vi "LaptopClient.vi"() -> ()   [LabVIEW 2018]
uses:
  Modes.ctl
  <vilib>/daq.io/MQTT LabVIEW Client/Controls/QoS.ctl
  <vilib>/daq.io/MQTT LabVIEW Client/Controls/DUP_Flag.ctl
  <vilib>/daq.io/MQTT LabVIEW Client/Controls/Retain_Flag.ctl
  <vilib>/daq.io/MQTT LabVIEW Client/Controls/Connect_Flags.ctl
  <vilib>/daq.io/MQTT LabVIEW Client/Controls/User_Info.ctl
  <vilib>/daq.io/MQTT LabVIEW Client/MQTT_Functions.lvlib
panel:
  out "Light":u16(ring)
  out "Fan":u16(ring)
  out "Reading Error":errorcluster
  out "Temperature":i32
  in  "Bulb":bool
  in  "Fan":bool
  in  "Mode Control":bool
  out "Mode":T1
  in  "stop":bool
  # "(auto)"
  # "(manual)"
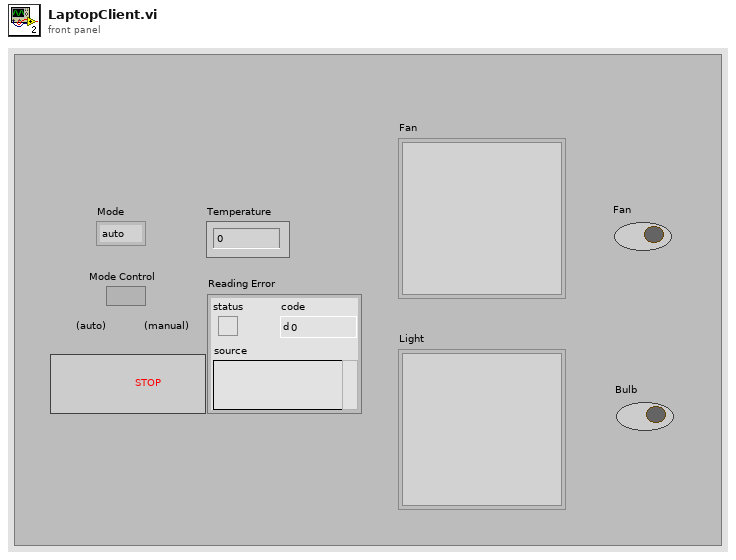
[diagram p1: front panel]
types:
  T1 = typedef "Modes.ctl" = enum16{"auto", "manual"}
  T2 = typedef "MQTT_Functions.lvlib/User_Info.ctl" = cluster{"User Name":string, "Password":string}
  T3 = typedef "MQTT_Functions.lvlib/QoS.ctl" = enum8{"At most once", "At least once", "Exactly once", "Reserved"}
  T4 = typedef "MQTT_Functions.lvlib/Connect_Flags.ctl" = cluster{"user name":bool, "password":bool, "will retain":bool, "will flag":bool, "clean session":bool, "reserved":bool, "will QoS":T3}
  T5 = typedef "MQTT_Functions.lvlib/DUP_Flag.ctl" = bool
  T6 = typedef "MQTT_Functions.lvlib/Retain_Flag.ctl" = bool
  T7 = cluster{"QoS":T3, "DUP":T5, "Retain":T6, "Keep Alive (sec)":u16}
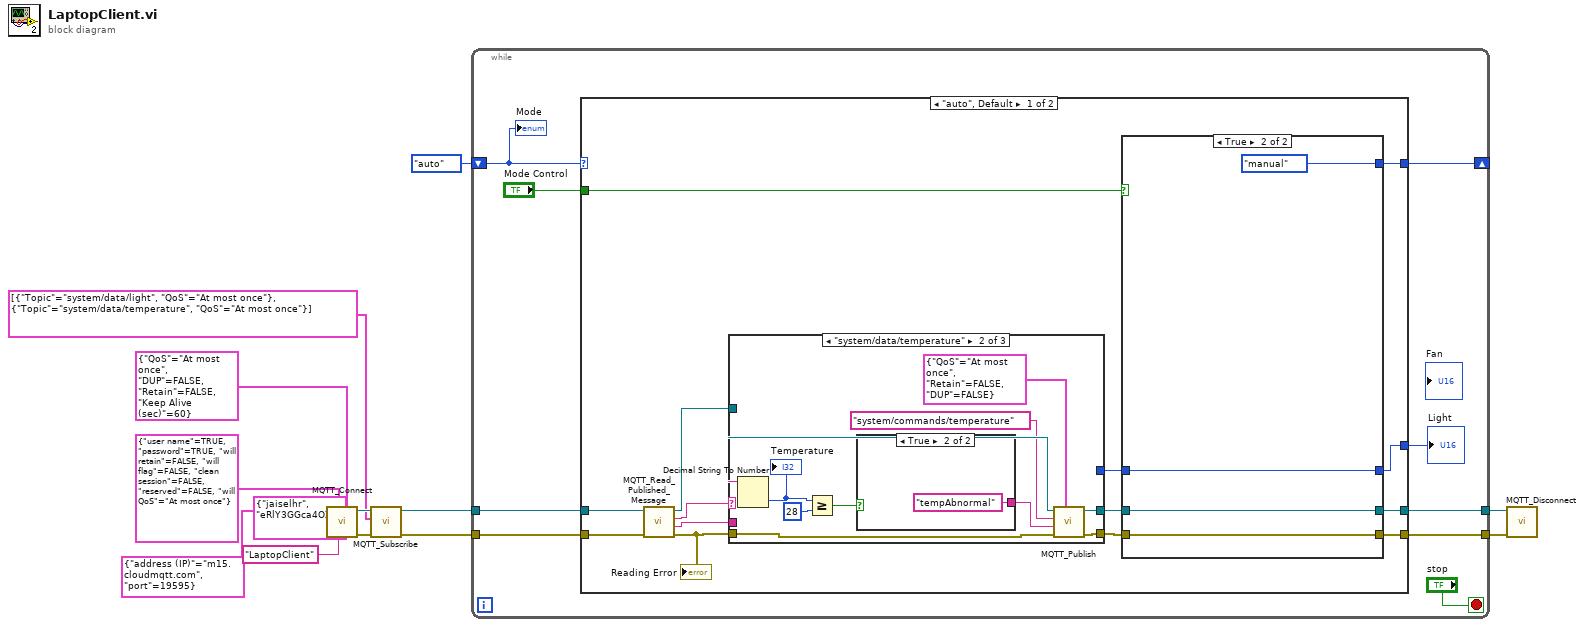
[diagram p0: block diagram]
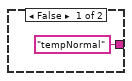
[diagram p3: hidden frame]
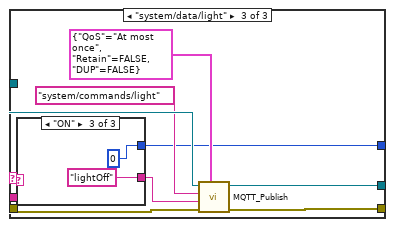
[diagram p4: hidden frame]
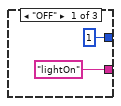
[diagram p5: hidden frame]
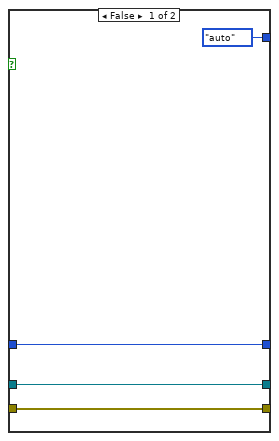
[diagram p7: hidden frame]
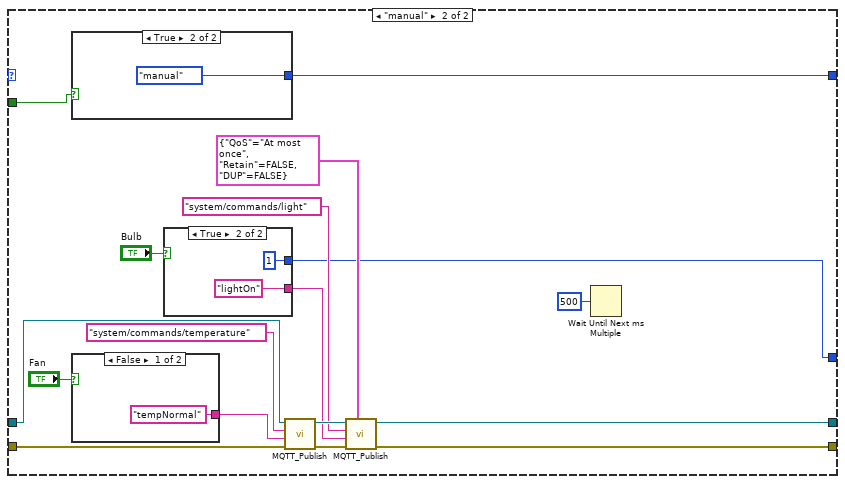
[diagram p8: hidden frame]
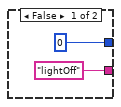
[diagram p9: hidden frame]
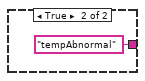
[diagram p10: hidden frame]
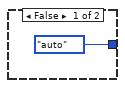
[diagram p11: hidden frame]
diagram:
  n1 = call <vilib>:"MQTT_Connect.vi"("Connect Meta"=T7 {"QoS"=enum."At most once", "DUP"=FALSE, "Retain"=FALSE, "Keep Alive (sec)"=60}, "Client ID"="LaptopClient", "Connect Flags"=T4 {"user name"=TRUE, "password"=TRUE, "will retain"=FALSE, "will flag"=FALSE, "clean session"=FALSE, "reserved"=FALSE, "will QoS"=enum."At most once"}, "User Info"=T2 {"User Name"="jaiselhr", "Password"="eRlY3GGca4OZ"}, "MQTT Broker"=cluster{"address (IP)":string, "port":u16} {"address (IP)"="m15.cloudmqtt.com", "port"=19595}) -> ("error out"=w7:errorcluster, "connection ID out"=w8:refnum<k5>)  [unwired: 4 in, 1 out]
  n2 = call <vilib>:"MQTT_Subscribe.vi"("error in (no error)"=w7, "Subscription Info Array"=cluster{"Topic":string, "QoS":T3}[] [{"Topic"="system/data/light", "QoS"=enum."At most once"}, {"Topic"="system/data/temperature", "QoS"=enum."At most once"}], "connection ID"=w8) -> ("error out"=w5:errorcluster, "connection ID out"=w4:refnum<k5>)  [unwired: 7 in]
  n3 = while {
    shift-right: [w21] -> _
    shift-left: Modes."auto" -> [w15]
    tunnel: w5 -> [w19]
    tunnel: w4 -> [w18]
    tunnel: [w17] -> w2
    tunnel: [w16] -> w3
    stop <- "stop" stop-if-true
    n4 = case shown="\"auto\", Default" w15 {
      tunnel: [w36 w88] -> w21
      tunnel: "Mode Control" -> [w35 w89]
      tunnel: w19 -> [w34 w84]
      tunnel: w18 -> [w33 w85]
      tunnel: [w26 w76] -> w17
      tunnel: [w25 w75] -> w16
      tunnel: [w23 w73] -> w14
      frame "auto", Default {
        n5 = call <vilib>:"MQTT_Read_Published_Message.vi"("error in (no error)"=w34, "connection ID"=w33) -> ("error out"=w30:errorcluster, "Message"=w31:string, "Topic Name"=w32:string, "connection ID out"=w28:refnum<k5>)  [unwired: 4 in, 2 out]
        "Reading Error" <- w30
        n6 = case shown="\"system/data/temperature\"" w32 {
          tunnel: w31 -> [_ w49 w60]
          tunnel: w30 -> [w38 w45 w59]
          tunnel: [w38 w44 w53] -> w29
          tunnel: w28 -> [w37 w41 w57]
          tunnel: [w37 w42 w56] -> w27
          tunnel: [_ _ w52] -> w24
          frame "False", Default {
          }
          frame "system/data/temperature" {
            n7 = Decimal String To Number(string=w49) -> (number=w48:i32)  [unwired: 2 in, 1 out]
            "Temperature" <- w48
            n8 = Greater Or Equal?(x=w48, y=28) -> (x >= y?=w46:bool)
            n9 = case shown="True" w46 {
              tunnel: ["tempNormal" ("Message to be published") "tempAbnormal" ("Message to be published")] -> w43
              frame False {
              }
              frame True {
              }
            }
            n10 = call <vilib>:"MQTT_Publish.vi"("Publish Meta"=cluster{"QoS":T3, "Retain":T6, "DUP":T5} {"QoS"=enum."At most once", "Retain"=FALSE, "DUP"=FALSE}, "error in (no error)"=w45, "Message to be published"=w43, "Topic"="system/commands/temperature", "connection ID"=w41) -> ("error out"=w44:errorcluster, "connection ID out"=w42:refnum<k5>)  [unwired: 5 in]
          }
          frame "system/data/light" {
            n11 = case shown="\"ON\"" w60 {
              tunnel: ["lightOn" ("Message to be published") _ "lightOff" ("Message to be published")] -> w58
              tunnel: [u16 1 ("Light") _ u16 0 ("Light")] -> w52
              frame "OFF" {
              }
              frame "", Default {
              }
              frame "ON" {
              }
            }
            n12 = call <vilib>:"MQTT_Publish.vi"("Publish Meta"=cluster{"QoS":T3, "Retain":T6, "DUP":T5} {"QoS"=enum."At most once", "Retain"=FALSE, "DUP"=FALSE}, "error in (no error)"=w59, "Message to be published"=w58, "Topic"="system/commands/light", "connection ID"=w57) -> ("error out"=w53:errorcluster, "connection ID out"=w56:refnum<k5>)  [unwired: 5 in]
          }
        }
        n13 = case shown="True" w35 {
          tunnel: [Modes."auto" ("Enum") Modes."manual" ("Enum")] -> w36
          tunnel: w29 -> [w66 w70]
          tunnel: w27 -> [w67 w71]
          tunnel: [w67 w71] -> w26
          tunnel: [w66 w70] -> w25
          tunnel: w24 -> [w65 w69]
          tunnel: [w65 w69] -> w23
          frame False {
          }
          frame True {
          }
        }
      }
      frame "manual" {
        n14 = case shown="True" w89 {
          tunnel: [Modes."auto" ("Enum") Modes."manual" ("Enum")] -> w88
          frame False {
          }
          frame True {
          }
        }
        n15 = case shown="False" "Fan" {
          tunnel: ["tempNormal" ("Message to be published") "tempAbnormal" ("Message to be published")] -> w83
          frame False {
          }
          frame True {
          }
        }
        n16 = case shown="True" "Bulb" {
          tunnel: ["lightOff" ("Message to be published") "lightOn" ("Message to be published")] -> w79
          tunnel: [u16 0 ("Light") u16 1 ("Light")] -> w73
          frame False {
          }
          frame True {
          }
        }
        n17 = call <vilib>:"MQTT_Publish.vi"("error in (no error)"=w84, "Message to be published"=w83, "Topic"="system/commands/temperature", "connection ID"=w85) -> ("error out"=w80:errorcluster, "connection ID out"=w81:refnum<k5>)  [unwired: 6 in]
        n18 = call <vilib>:"MQTT_Publish.vi"("Publish Meta"=cluster{"QoS":T3, "Retain":T6, "DUP":T5} {"QoS"=enum."At most once", "Retain"=FALSE, "DUP"=FALSE}, "error in (no error)"=w80, "Message to be published"=w79, "Topic"="system/commands/light", "connection ID"=w81) -> ("error out"=w75:errorcluster, "connection ID out"=w76:refnum<k5>)  [unwired: 5 in]
        n19 = Wait Until Next ms Multiple(millisecond multiple=u32 500) -> ()  [unwired: 1 out]
      }
    }
    "Light" <- w14
    "Mode" <- w15
  }
  n20 = call <vilib>:"MQTT_Disconnect.vi"("error in (no error)"=w3, "connection ID"=w2) -> ()  [unwired: 9 in, 1 out]
